vi "Close.vi"(8 "error in (no error)":errorcluster, 11 "FW102C in":i32) -> (0 "error out":errorcluster)   [LabVIEW 2018, in "Thorlabs_FW102C.lvlib"]
uses:
  Thorlabs_FW102C.lvlib
  <instrlib>/Thorlabs_FW102C/Library/FilterWheel102_win32.dll
  Library/FilterWheel102_win64.dll
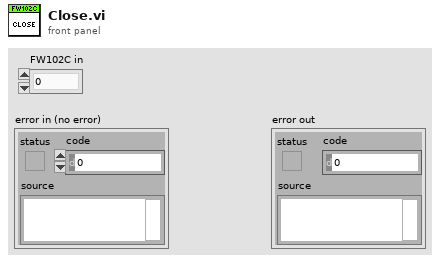
[diagram p1: front panel]
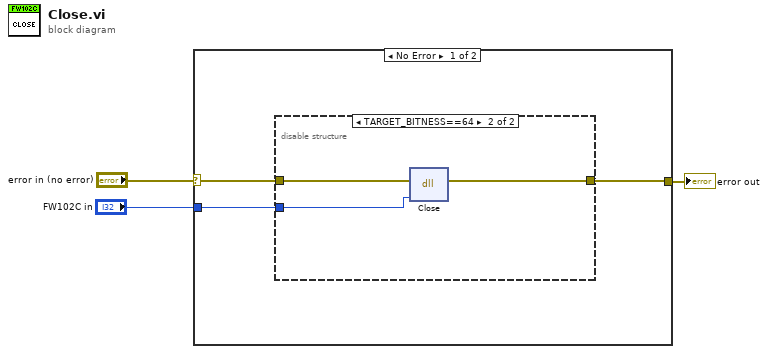
[diagram p0: block diagram]
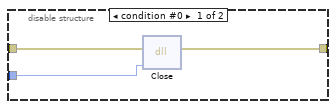
[diagram p2: hidden frame]
diagram:
  n1 = case shown="No Error" "error in (no error)" {
    selector: "error in (no error)" -> [w6 w13]
    tunnel: [w5 w13] -> w2
    tunnel: "FW102C in" -> [w4 _]
    frame No Error {
      n2 = disable-structure shown="TARGET_BITNESS==64" {
        disable-tunnel: w6 -> [w9 w12]
        disable-tunnel: [w8 w11] -> w5
        disable-tunnel: w4 -> [w7 w10]
        frame condition #0 {
          n3 = dll-call lib="E:/Program Files (x86)/National Instruments/LabVIEW 2011/instr.lib/Thorlabs_FW102C/Library/FilterWheel102_win32.dll" fn="Close"(error in=w9, "hdl"=w7) -> (error out=w8:errorcluster)  [unwired: 4 in, 1 out]
        }
        frame condition #1 (active) {
          n4 = dll-call lib="C:/Users/aspitarl/Git/MHDlab/Instruments/Not Updated Yet/Filter Wheel/Thorlabs_FW102C/Library/FilterWheel102_win64.dll" fn="Close"(error in=w12, "hdl"=w10) -> (error out=w11:errorcluster)  [unwired: 4 in, 1 out]
        }
      }
    }
    frame Error {
    }
  }
  "error out" <- w2
